vi "stimulus.vi"(7 "幅值(V)":dbl, 8 "stop frequency [Hz]":dbl, 9 "start frequency [Hz]":dbl, 10 "信号时长":dbl, 11 "Format":cluster{"Rate":i32, "Bits":i32, "Channels":u32}={"Rate"=44100, "Bits"=32, "Channels"=2}) -> (0 "sti":dbl[](array[numeric]), 2 "Buffer size":i32, 3 "Output data":i32[][](array[numeric]))   [LabVIEW 2021]
uses:
  Global.vi
  <vilib>/measure/NI_MABase.lvlib
  <vilib>/addons/_NISVFA/_Generation/SoundVib_Generation.lvlib
panel:
  in  "信号时长(s)":dbl
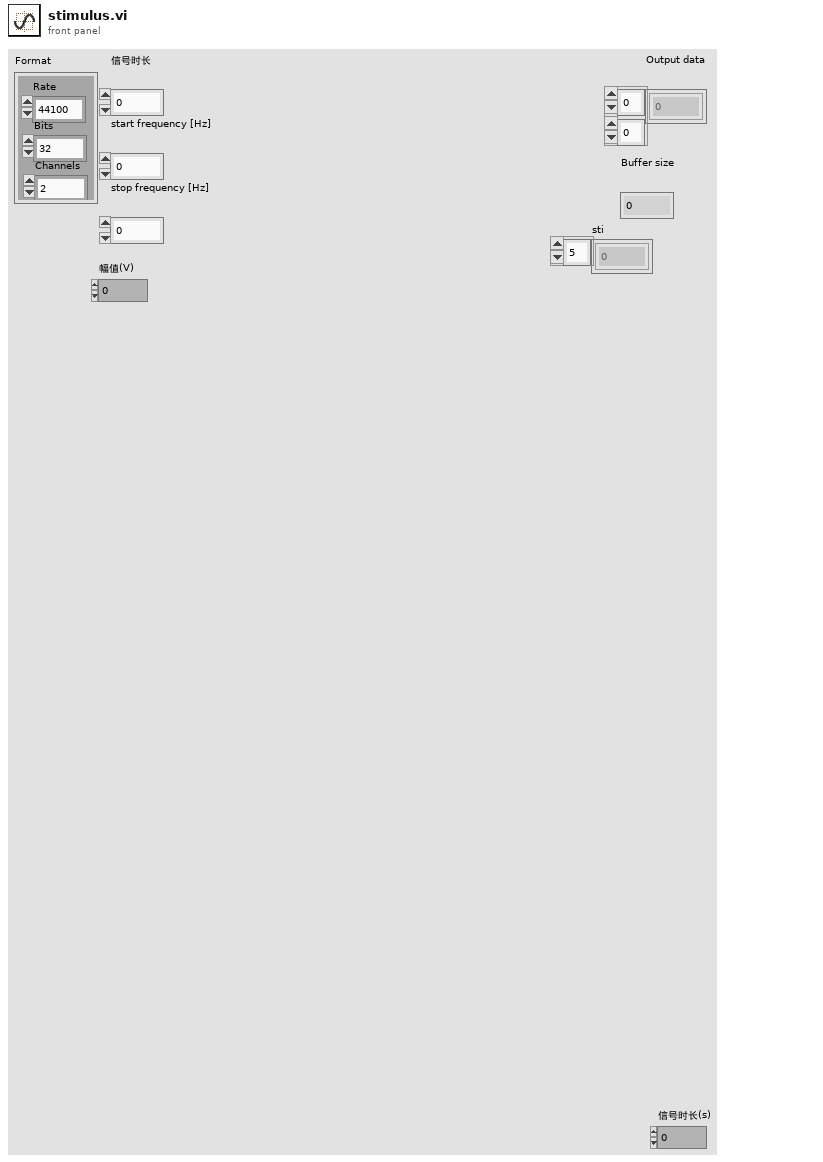
[diagram p1: front panel]
types:
  T1 = cluster{"start frequency [Hz]":dbl, "stop frequency [Hz]":dbl}
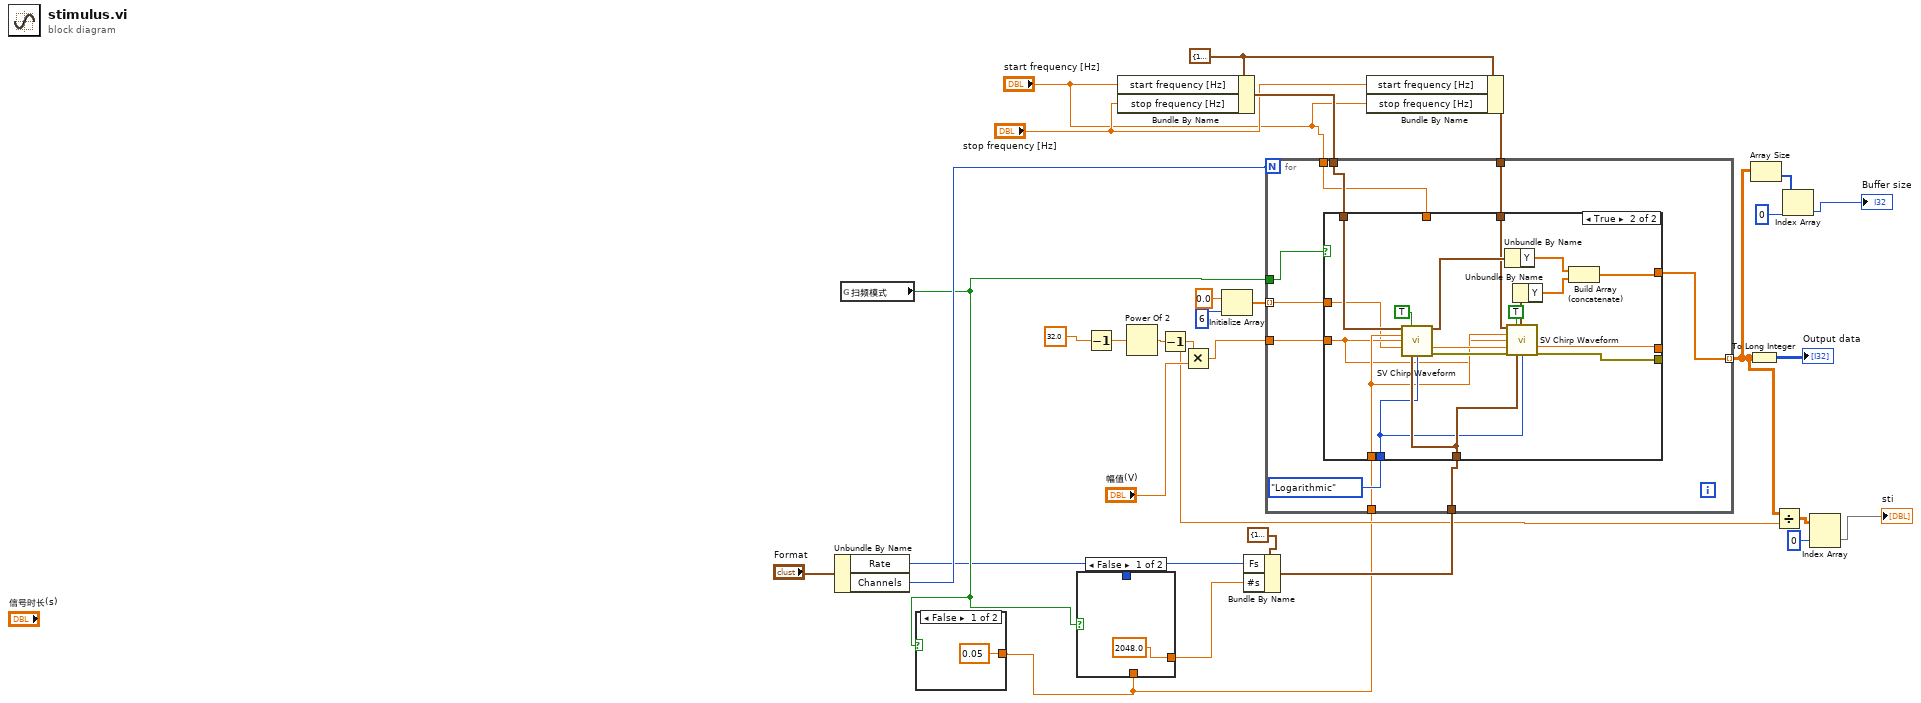
[diagram p0: block diagram]
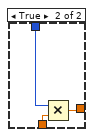
[diagram p2: hidden frame]
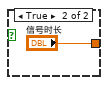
[diagram p3: hidden frame]
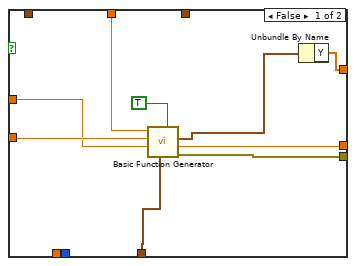
[diagram p4: hidden frame]
diagram:
  w11 = T1 {"start frequency [Hz]"=10.0, "stop frequency [Hz]"=10000.0} ("frequency range")
  n1 = Unbundle By Name("Format") -> ("Rate"=w12:i32, "Channels"=w20:u32)
  n2 = global read "Global.vi" "扫频模式"() -> (w14:bool)
  n3 = case shown="False" w14 {
    tunnel: [0.05 ("信号时长") "信号时长"] -> w7
    frame False {
    }
    frame True {
    }
  }
  n4 = case shown="False" w14 {
    tunnel: [2048.0 w36] -> w13
    tunnel: w7 -> [_ w34]
    tunnel: w12 -> [_ w35]
    frame False {
    }
    frame True {
      n5 = Multiply(x=w35, y=w34) -> (x*y=w36:dbl)
    }
  }
  n6 = Decrement(x=32.0) -> (x-1=w27:dbl)
  n7 = Bundle By Name(cluster=w11, "start frequency [Hz]"="start frequency [Hz]", "stop frequency [Hz]"="stop frequency [Hz]") -> (w22:T1)
  n8 = Power Of 2(x=w27) -> (2^x=w26:dbl)
  n9 = Decrement(x=w26) -> (x-1=w21:dbl)
  n10 = Multiply(x=w21, y="幅值(V)") -> (x*y=w29:dbl)
  n11 = Initialize Array(0.0 ("element"), 6 ("dimension size")) -> (w4:dbl[])
  n12 = Bundle By Name(cluster=cluster{"Fs":dbl, "#s":dbl} {"Fs"=1000.0, "#s"=1000.0} ("sampling info"), "Fs"=w12, "#s"=w13) -> (w23:cluster{"Fs":dbl, "#s":dbl})
  n13 = Bundle By Name(cluster=w11, "start frequency [Hz]"="stop frequency [Hz]", "stop frequency [Hz]"="start frequency [Hz]") -> (w8:T1)
  n14 = for {
    N: w20 -> [_]
    tunnel: w29 -> [w40]
    tunnel: w23 -> [w45]
    tunnel: w22 -> [w43]
    tunnel: w14 -> [w44]
    tunnel: "start frequency [Hz]" -> [w38]
    tunnel: w8 -> [w42]
    tunnel: w7 -> [w41]
    tunnel: w4 -> [w39] mode=indexing
    tunnel: [w37] -> w1 mode=indexing
    n15 = case shown="True" w44 {
      tunnel: w45 -> [w54 w63]
      tunnel: enum16{"Linear", "Logarithmic"}."Logarithmic" ("frequency spacing") -> [_ w62]
      tunnel: [w55 w72] -> _
      tunnel: [w53 w68] -> _
      tunnel: [w51 w56] -> w37
      tunnel: w43 -> [_ w61]
      tunnel: w42 -> [_ w60]
      tunnel: w41 -> [_ w59]
      tunnel: w40 -> [w48 w58]
      tunnel: w39 -> [w47 w57]
      tunnel: w38 -> [w49 _]
      frame False {
        n16 = call <vilib>:"Basic Function Generator.vi"("reset signal"=TRUE, "sampling info"=w54, "phase"=w47, "amplitude"=w48, "frequency"=w49) -> ("error out"=w55:errorcluster, "phase out"=w53:dbl, "signal out"=w52:waveform(dbl))  [unwired: 4 in]
        n17 = Unbundle By Name(w52) -> ("Y"=w51:dbl[])
      }
      frame True {
        n18 = call <vilib>:"SV Chirp Waveform.vi"("frequency range"=w61, "reset signal (F)"=TRUE, "chirp duration [s]"=w59, "amplitude"=w58, "phase in [deg]"=w57, "sampling info"=w63, "frequency spacing"=w62) -> ("chirp signal"=w67:waveform(dbl), "phase out [deg]"=w70:dbl, "error out"=w72:errorcluster)  [unwired: 6 in]
        n19 = Unbundle By Name(w67) -> ("Y"=w65:dbl[])
        n20 = call <vilib>:"SV Chirp Waveform.vi"("frequency range"=w60, "reset signal (F)"=TRUE, "chirp duration [s]"=w59, "amplitude"=w58, "phase in [deg]"=w70, "sampling info"=w63, "frequency spacing"=w62) -> ("chirp signal"=w66:waveform(dbl), "phase out [deg]"=w68:dbl)  [unwired: 6 in, 1 out]
        n21 = Unbundle By Name(w66) -> ("Y"=w64:dbl[])
        n22 = Build Array (concatenate)(w65, w64) -> (w56:dbl[])
      }
    }
  }
  n23 = To Long Integer(number=w1) -> (32bit integer=→"Output data":i32[][])
  n24 = Array Size(array=w1) -> (size(s)=w18:i32[])
  n25 = Divide(x=w1, y=w21) -> (x/y=w3:dbl[][])
  n26 = Index Array(array=w18, index=0) -> (element=→"Buffer size":i32)
  n27 = Index Array(array=w3, index (row)=0) -> (element=→"sti":dbl[])  [unwired: 1 in]
